vi "Actor Core.vi"(8 "error in":errorcluster, 11 "Nested in":refnum<class "CameraController.lvclass">) -> (0 "error out":errorcluster, 3 "Actor out":refnum<class "Actor.lvclass">)   [LabVIEW 2020, in "CameraController.lvlib" / "CameraController.lvclass"]
doc: "(<B>Filename</B>: Actor Framework.lvlib:Actor.lvclass:Actor Core.vi)\n\nReceives messages to the actor, reacts to them, and initiates any error handling that may shut the actor down.\n\nDescendant classes may override this VI to append parallel tasks for the actor to complete while it handles messages. Overrides use the Call Parent Method node."
uses:
  CameraController.lvclass
  <vilib>/ActorFramework/Actor/Actor.lvclass
  <vilib>/ActorFramework/Stop Msg/Stop Msg.lvclass
  C:/Program Files/National Instruments/LabVIEW 2020/vi.lib/ActorFramework/Actor/Actor.lvclass
  D:/Daguan/Development/MMicroscopyFramework/ViewController/Prime95BCameraController/CameraController.lvclass
  D:/Daguan/Development/MMicroscopyFramework/Interface/DataListener/DataListener.lvclass
  Model/Hardware Abstraction Layer/Component/Camera/Camera Messages/SetExposure Msg/SetExposure Msg.lvclass
  Model/Hardware Abstraction Layer/Component/Device/Device Messages/StopAcquisition Msg/StopAcquisition Msg.lvclass
  Model/Hardware Abstraction Layer/Component/Camera/Camera Messages/SetBinning Msg/SetBinning Msg.lvclass
  Interface/StageController Messages/SetStagePosition Msg/SetStagePosition Msg.lvclass
  Model/Hardware Abstraction Layer/Component/Camera/Camera Messages/SetFrameToCaptureNumber Msg/SetFrameToCaptureNumber Msg.lvclass
  Model/Hardware Abstraction Layer/Component/Camera/Camera Messages/SetInterval Msg/SetInterval Msg.lvclass
  CameraController Messages/PrepareAndSendROI Msg/PrepareAndSendROI Msg.lvclass
  Model/Hardware Layer/Real Hardware/Camera_Prime95B/Camera_Prime95B/Controls/Camera Status.ctl
  Model/Hardware Layer/Real Hardware/Camera_Prime95B/Camera_Prime95B/Camera_Prime95B.lvclass
  CameraController Messages/PrepareAndSendStartAcq Msg/PrepareAndSendStartAcq Msg.lvclass
panel:
  in  "Display?":bool
  in  "ThreadholdMin":i32=500
  in  "ROITool":bool
  in  "ZoomTool":bool
  in  "Autostretch":bool
  in  "ZoomToFit":bool
  in  "Save Path":path
  in  "Alert when finish?":bool
  in  "SingleStack?":bool
  in  "StreamToDisk?":bool
  in  "Binning":enum32{"1x1", "2x2"}(radio)
  in  "File Suffix":string
  in  "Full":bool
  in  "Crop":bool
  in  "Scale Bar":bool
  in  "ScaleBarSize":dbl caption="um" min=0.0 max=50.0
  in  "ThreadholdMax":u32(slide) max=4096 step=1 scale=0.0..10.0
  in  "Save Settings":bool
  in  "Snap":bool
  in  "Live":bool
  in  "Acquire":bool
  in  "Stop":bool
  in  "Album":bool
  in  "Exit":bool
  in  "Interval":dbl min=0.0 max=99999.0
  in  "Frames":dbl min=0.0 max=5000.0
  in  "ExposureMs":dbl min=0.0 max=99999.0
  out "DropFrames":dbl
  out "RealFPS":dbl
  out "ImgIndex":dbl
  out "RawImage":T1(plugin-control)
  # "ROI"
  # "Save Image Mode"
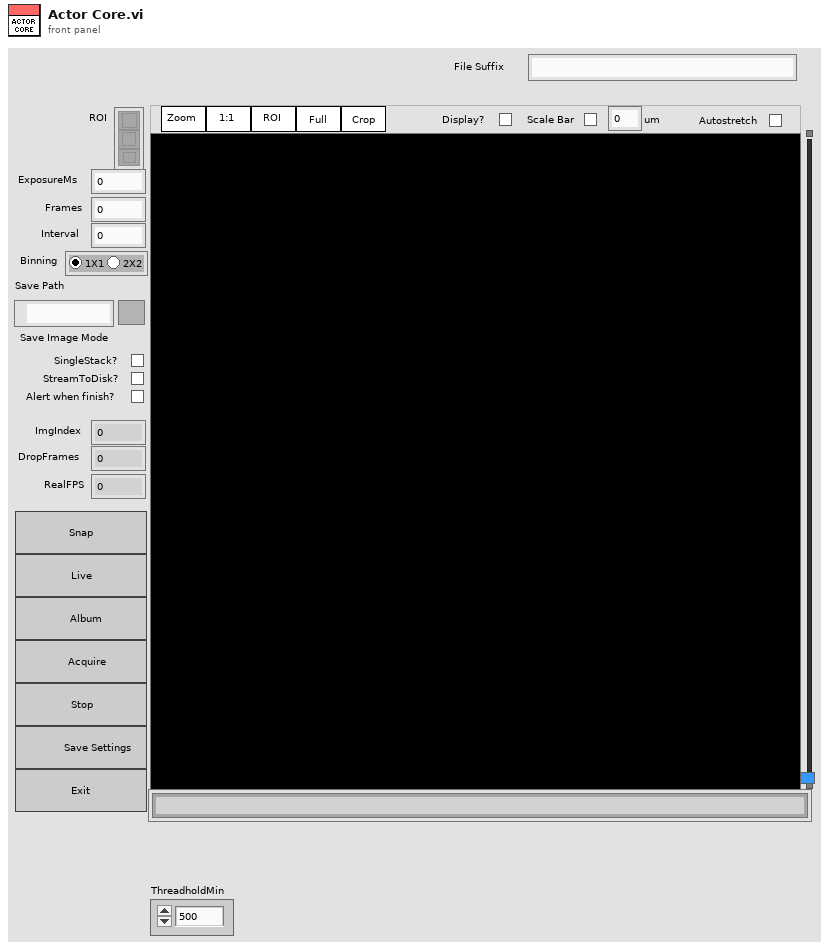
[diagram p1: front panel]
types:
  T1 = typedef "IMAQ Image.ctl" = refnum<image>
  T2 = cluster{"Stop":refnum<user-event>, "RawImage":refnum<user-event>}
  T3 = cluster{"Global Rectangle":i32[], "Contours":cluster{"Contour Type":u32, "ROI Type":u32, "Points":i32[]}[]}
  T4 = typedef "Camera_Prime95B.lvlib/Camera_Prime95B.lvclass/Camera Status.ctl" = i32
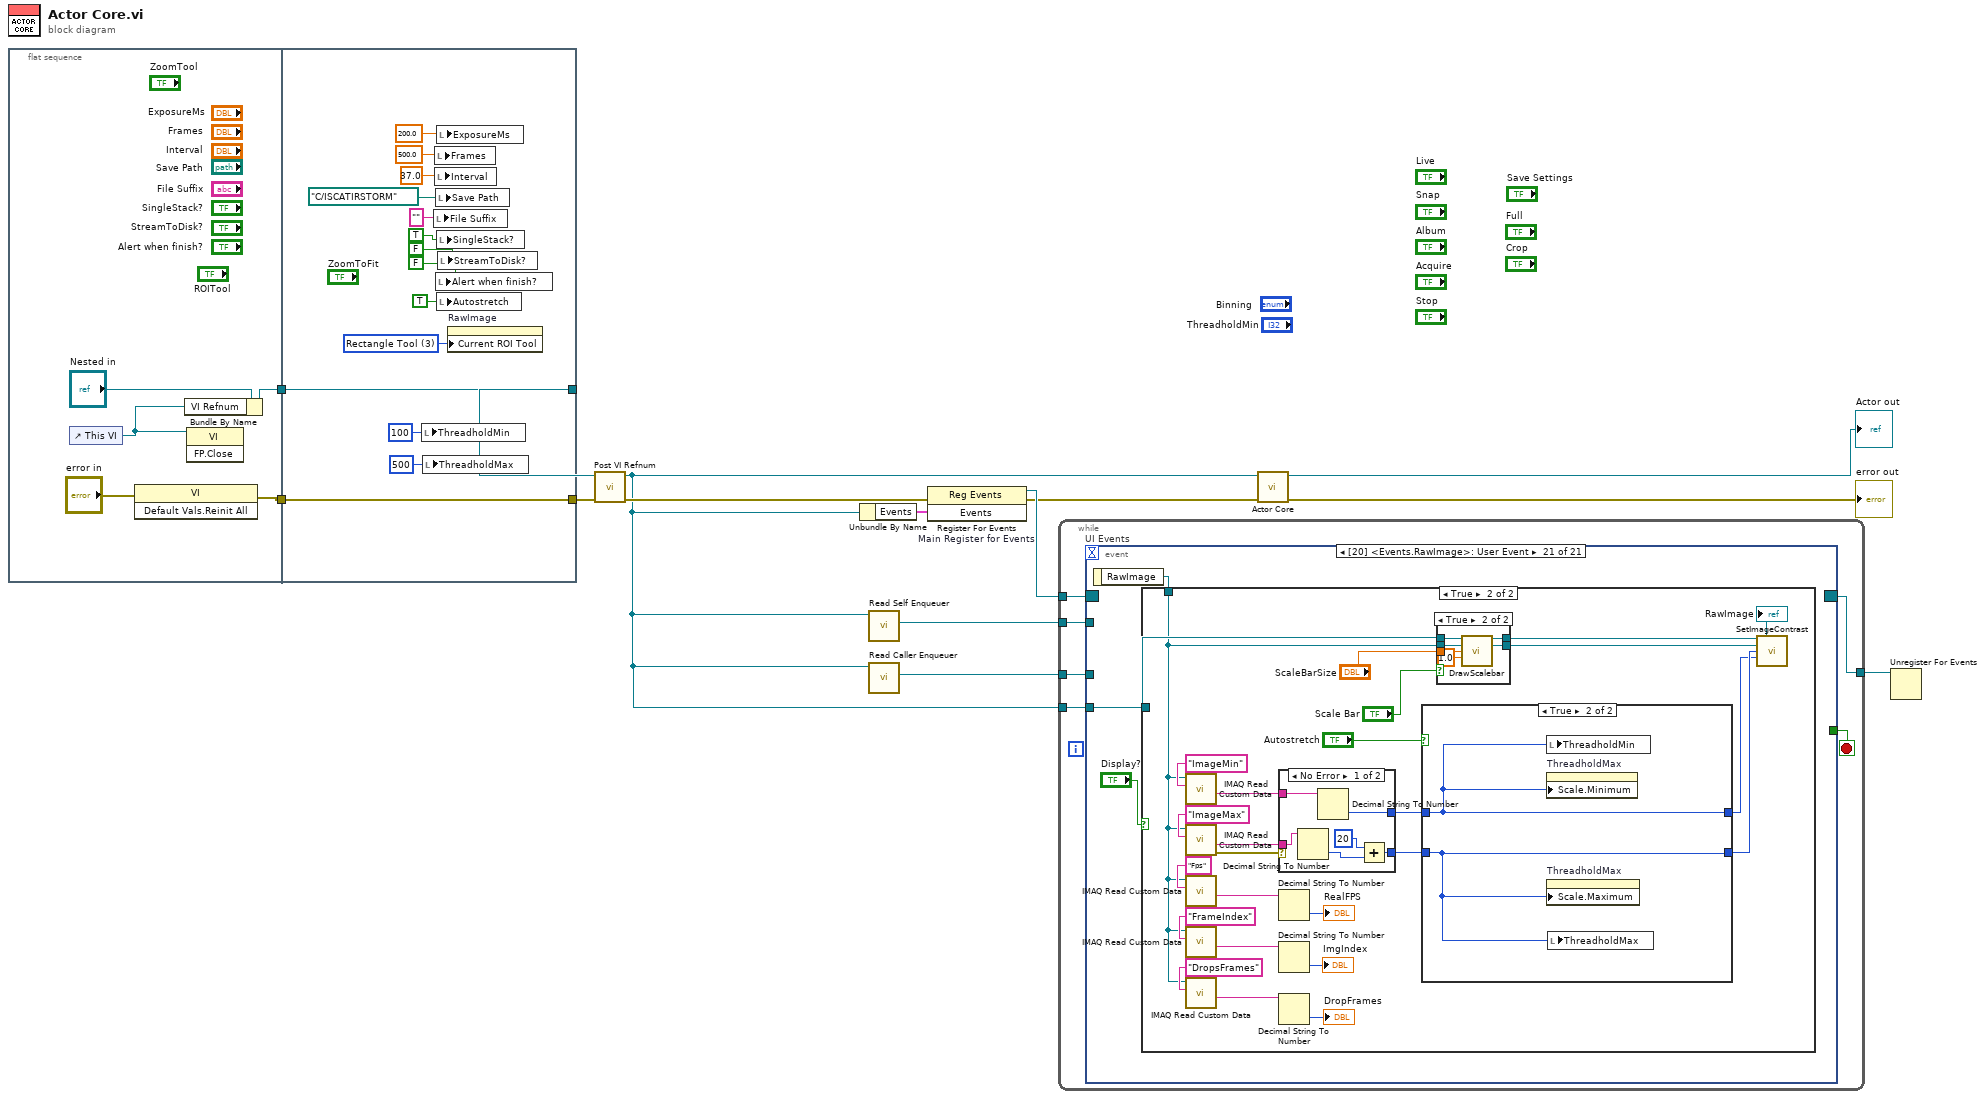
[diagram p0: block diagram]
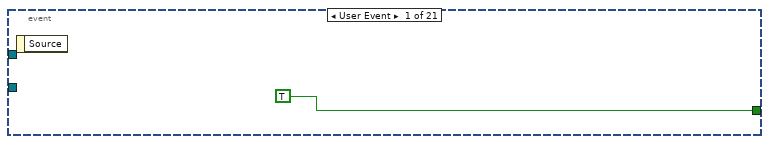
[diagram p2: hidden frame]
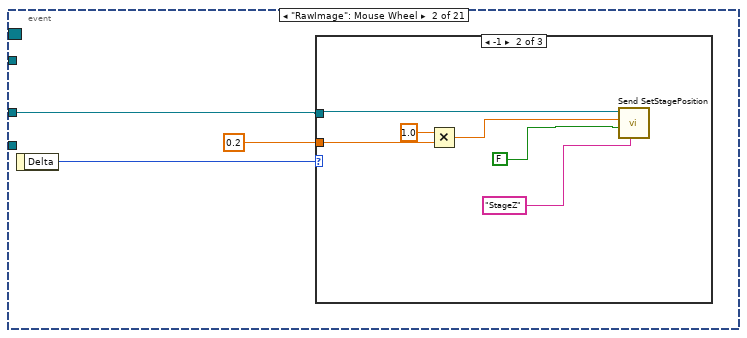
[diagram p3: hidden frame]
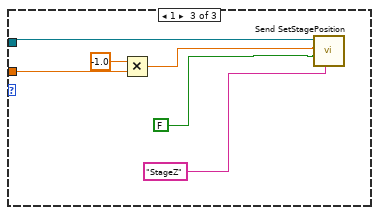
[diagram p5: hidden frame]
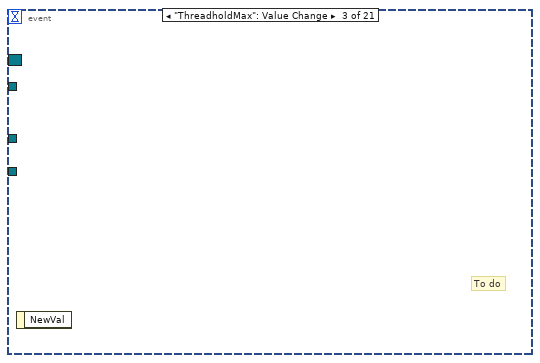
[diagram p6: hidden frame]
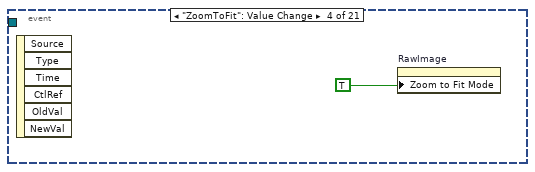
[diagram p7: hidden frame]
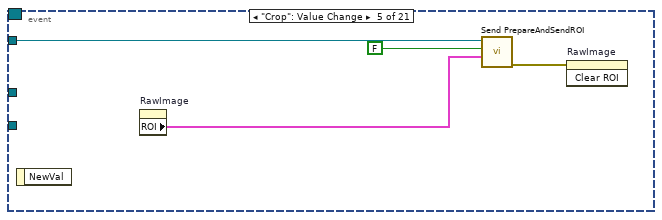
[diagram p8: hidden frame]
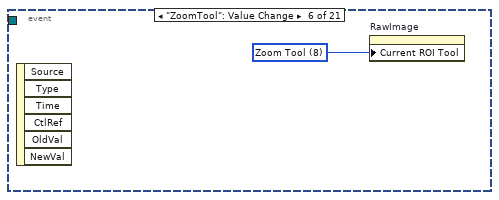
[diagram p9: hidden frame]
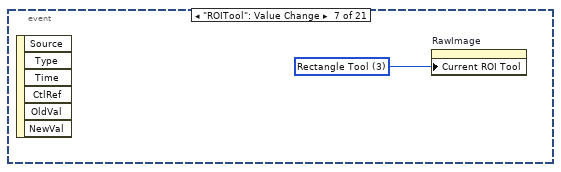
[diagram p10: hidden frame]
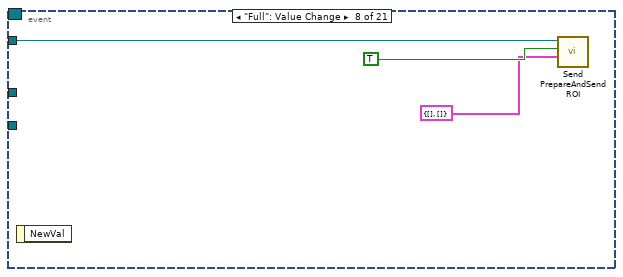
[diagram p11: hidden frame]
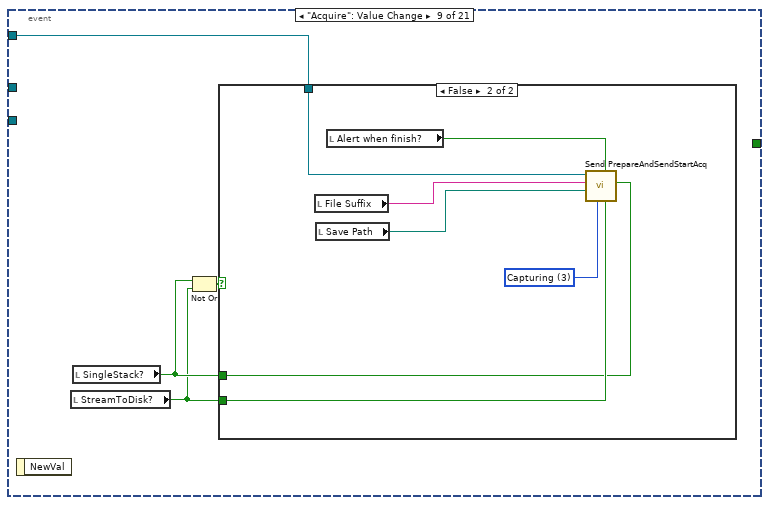
[diagram p12: hidden frame]
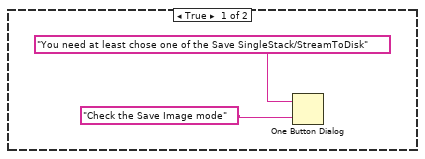
[diagram p13: hidden frame]
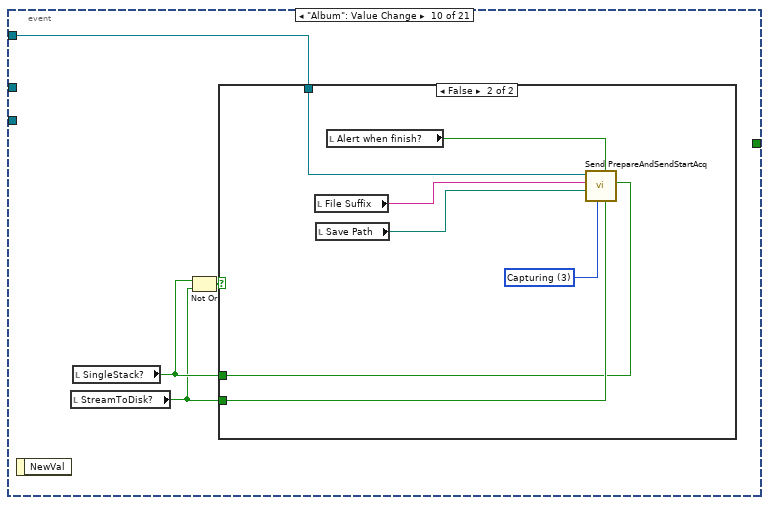
[diagram p14: hidden frame]
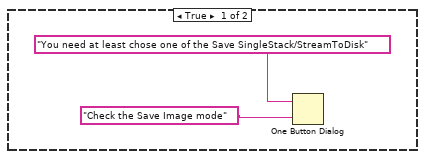
[diagram p15: hidden frame]
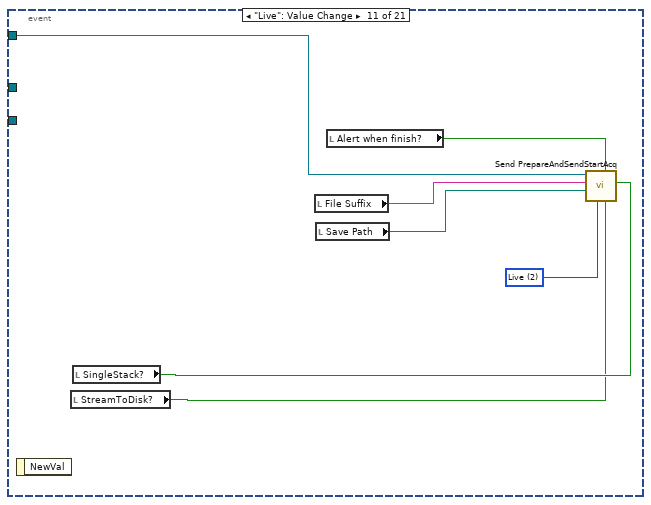
[diagram p16: hidden frame]
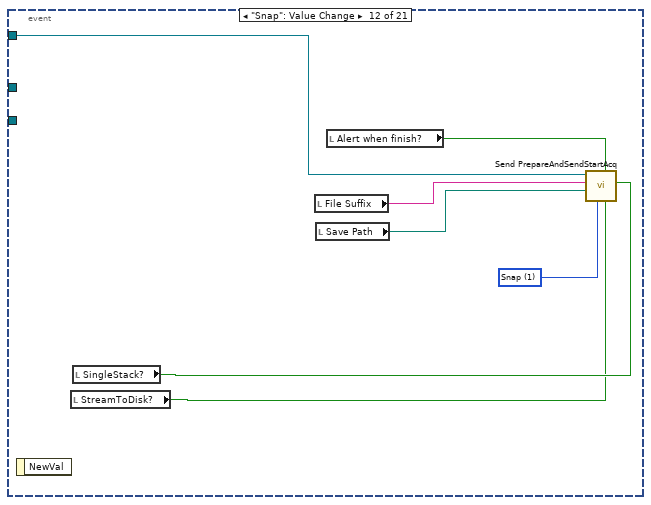
[diagram p17: hidden frame]
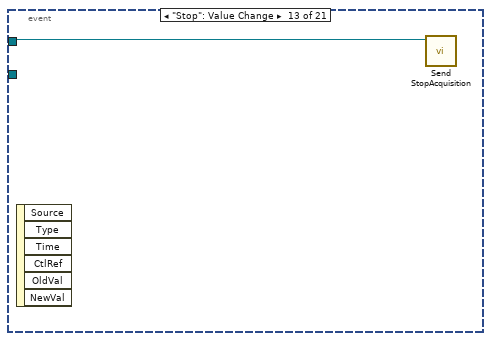
[diagram p18: hidden frame]
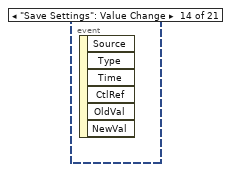
[diagram p19: hidden frame]
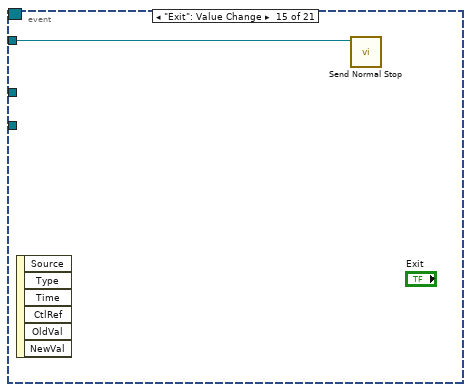
[diagram p20: hidden frame]
diagram:
  n1 = flat-sequence {
    tunnel: [w17] -> w6
    tunnel: [w16] -> w5
    tunnel: [w32] -> w2
    tunnel: [w33] -> w7
    tunnel: w6 -> [w33]
    tunnel: w5 -> [w32]
    frame #0 {
      n2 = control-ref of="This VI"() -> (w15:refnum<vi>)
      n3 = invoke class="VI" method="Default Vals.Reinit All"(error in="error in") -> (error out=w17:errorcluster)  [unwired: 2 in, 2 out]
      n4 = Bundle By Name(cluster="Nested in", "VI Refnum"=w15) -> (w16:refnum<class "CameraController.lvclass">)
      n5 = invoke class="VI" method="FP.Close"(reference=w15) -> ()  [unwired: 2 in, 3 out]
    }
    frame #1 {
      w23 = u32 3 items=["Zoom Tool"=8, "Selection Tool"=0, "Pan Tool"=9, "Point Tool"=1, "Line Tool"=2, "Rectangle Tool"=3, "Rotated Rectangle Tool"=12, "Polyline Tool"=10, "Polygon Tool"=5, "Freehand Tool"=11, "Closed Freehand Tool"=6, "Ellipse Tool"=4, "Annulus Tool"=7] ("Current ROI Tool")
      n6 = local write "ThreadholdMin"(100 ("ThreadholdMin")) -> ()
      n7 = local write "ThreadholdMax"(u32 500 ("ThreadholdMax")) -> ()
      n8 = local write "File Suffix"("" ("File suffix")) -> ()
      n9 = local write "Frames"(500.0 ("Frames")) -> ()
      n10 = local write "Interval"(37.0 ("Interval")) -> ()
      n11 = local write "Save Path"(path "C:/ISCATIRSTORM" ("Save Path")) -> ()
      n12 = local write "Alert when finish?"(FALSE ("Alert when finish?")) -> ()
      n13 = local write "ExposureMs"(200.0 ("ExposureMs")) -> ()
      n14 = local write "SingleStack?"(TRUE ("SingleStack?")) -> ()
      n15 = local write "Autostretch"(TRUE ("Autostretch")) -> ()
      n16 = local write "StreamToDisk?"(FALSE ("StreamToDisk?")) -> ()
      n17 = property on="RawImage" class="ImageControl"("Current ROI Tool"=w23) -> ()  [unwired: 2 in, 2 out]
    }
  }
  n18 = call-dynamic "Post VI Refnum.vi"("error in (no error)"=w7, "Camera Prime95B Controller in"=w2) -> ("error out"=w3:errorcluster, "Camera Prime95B Controller out"=w1:refnum<class "CameraController.lvclass">)  [unwired: 8 in]
  n19 = Unbundle By Name(w1) -> ("Events"=w11:T2)
  n20 = call <vilib>:"Read Self Enqueuer.vi"("Actor"=w1) -> ("Self Enqueuer"=w9:refnum<class "Message Enqueuer.lvclass">)  [unwired: 10 in]
  n21 = call <vilib>:"Read Caller Enqueuer.vi"("Actor"=w1) -> ("Caller Enqueuer"=w4:refnum<class "Message Enqueuer.lvclass">)  [unwired: 10 in]
  n22 = register-events "Main Register for Events"(error in=w3, w11) -> (reference out=w12:refnum<event-registration>, error out=w8:errorcluster)  [unwired: 1 in]
  n23 = while {
    tunnel: w12 -> [w39]
    tunnel: [w37] -> w10
    tunnel: w9 -> [w36]
    tunnel: w4 -> [w35]
    tunnel: w1 -> [w34]
    stop <- w38 stop-if-true
    n24 = event "UI Events" shown="[20] <Events.RawImage>: User Event" {
      selector: w39 -> [_ _ _ _ _ _ _ _ _ _ _ _ _ _ _ _ _ _ _ _ _]
      dyn-events: [_ _ _ _ _ _ _ _ _ _ _ _ _ _ _ _ _ _ _ _ _] -> w37
      timeout: _ -> [_ _ _ _ _ _ _ _ _ _ _ _ _ _ _ _ _ _ _ _ _]
      tunnel: [TRUE _ _ _ _ _ _ _ _ _ _ _ _ _ _ _ _ _ _ _ _] -> w38
      tunnel: w36 -> [_ _ _ _ w60 _ _ w65 w66 w79 w96 w103 _ _ w107 _ _ _ _ w117 _]
      tunnel: w35 -> [_ w42 _ _ _ _ _ _ _ _ _ _ w106 _ _ w109 w111 w113 w116 _ _]
      tunnel: w34 -> [_ _ _ _ _ _ _ _ _ _ _ _ _ _ _ _ _ _ _ _ w121]
      event User Event {
        n25 = event-data() -> ()  [unwired: 1 in, 1 out]
      }
      event "RawImage": Mouse Wheel {
        n26 = event-data() -> ("Delta"=w43:i32)  [unwired: 1 in]
        n27 = case shown="-1" w43 {
          tunnel: w42 -> [_ w47 w53]
          tunnel: 0.2 ("Value") -> [_ w49 w55]
          frame 0, Default {
          }
          frame -1 {
            n28 = Multiply(x=1.0, y=w49) -> (x*y=w46:dbl)
            n29 = call "Send SetStagePosition.vi"("Label"="StageZ" ("Message"), "AbsPosition?"=FALSE, "Value"=w46, "Message Enqueuer"=w47) -> ()  [unwired: 6 in, 2 out]
          }
          frame 1 {
            n30 = Multiply(x=-1.0, y=w55) -> (x*y=w52:dbl)
            n31 = call "Send SetStagePosition.vi"("Label"="StageZ" ("Message"), "AbsPosition?"=FALSE, "Value"=w52, "Message Enqueuer"=w53) -> ()  [unwired: 6 in, 2 out]
          }
        }
      }
      event "ThreadholdMax": Value Change {
        # "To do"
        n32 = event-data() -> ()  [unwired: 1 in, 1 out]
      }
      event "ZoomToFit": Value Change {
        n33 = event-data() -> ()  [unwired: 1 in, 6 out]
        n34 = property on="RawImage" class="ImageControl"("Zoom to Fit Mode"=TRUE) -> ()  [unwired: 2 in, 2 out]
      }
      event "Crop": Value Change {
        n35 = event-data() -> ()  [unwired: 1 in, 1 out]
        n36 = property on="RawImage" class="ImageControl"() -> ("ROI"=w58:T3)  [unwired: 2 in, 2 out]
        n37 = call "Send PrepareAndSendROI.vi"("ROI"=w58, "Clear ROI?(F)"=FALSE, "Message Enqueuer"=w60) -> ("error out"=w57:errorcluster)  [unwired: 7 in, 1 out]
        n38 = invoke on="RawImage" class="ImageControl" method="Clear ROI"(error in=w57) -> ()  [unwired: 2 in, 3 out]
      }
      event "ZoomTool": Value Change {
        w61 = u32 8 items=["Zoom Tool"=8, "Selection Tool"=0, "Pan Tool"=9, "Point Tool"=1, "Line Tool"=2, "Rectangle Tool"=3, "Rotated Rectangle Tool"=12, "Polyline Tool"=10, "Polygon Tool"=5, "Freehand Tool"=11, "Closed Freehand Tool"=6, "Ellipse Tool"=4, "Annulus Tool"=7] ("Current ROI Tool")
        n39 = event-data() -> ()  [unwired: 1 in, 6 out]
        n40 = property on="RawImage" class="ImageControl"("Current ROI Tool"=w61) -> ()  [unwired: 2 in, 2 out]
      }
      event "ROITool": Value Change {
        w62 = u32 3 items=["Zoom Tool"=8, "Selection Tool"=0, "Pan Tool"=9, "Point Tool"=1, "Line Tool"=2, "Rectangle Tool"=3, "Rotated Rectangle Tool"=12, "Polyline Tool"=10, "Polygon Tool"=5, "Freehand Tool"=11, "Closed Freehand Tool"=6, "Ellipse Tool"=4, "Annulus Tool"=7] ("Current ROI Tool")
        n41 = event-data() -> ()  [unwired: 1 in, 6 out]
        n42 = property on="RawImage" class="ImageControl"("Current ROI Tool"=w62) -> ()  [unwired: 2 in, 2 out]
      }
      event "Full": Value Change {
        n43 = event-data() -> ()  [unwired: 1 in, 1 out]
        n44 = call "Send PrepareAndSendROI.vi"("ROI"=T3 {"Global Rectangle"=[], "Contours"=[]}, "Clear ROI?(F)"=TRUE, "Message Enqueuer"=w65) -> ()  [unwired: 7 in, 2 out]
      }
      event "Acquire": Value Change {
        n45 = event-data() -> ()  [unwired: 1 in, 1 out]
        n46 = local read "StreamToDisk?"() -> (w68:bool)
        n47 = local read "SingleStack?"() -> (w69:bool)
        n48 = Not Or(1:w68, 2:w69) -> (0:w67:bool)
        n49 = case shown="False" w67 {
          tunnel: w69 -> [_ w72]
          tunnel: w68 -> [_ w74]
          tunnel: w66 -> [_ w78]
          frame True {
            n50 = One Button Dialog(message="You need at least chose one of the Save SingleStack/StreamToDisk", button name ("OK")="Check the Save Image mode" ("message")) -> ()  [unwired: 1 out]
          }
          frame False {
            w75 = T4 3 items=["Idle", "Snap", "Live", "Capturing", ""] ("Mode")
            n51 = local read "File Suffix"() -> (w77:string)
            n52 = local read "Save Path"() -> (w76:path)
            n53 = local read "Alert when finish?"() -> (w73:bool)
            n54 = call "Send PrepareAndSendStartAcq.vi"("SingleStack?"=w72, "StreamToDisk?"=w74, "Alert when finish?"=w73, "Mode"=w75, "Save Path"=w76, "File Suffix"=w77, "Message Enqueuer"=w78) -> ()  [unwired: 3 in, 2 out]
          }
        }
      }
      event "Album": Value Change {
        n55 = event-data() -> ()  [unwired: 1 in, 1 out]
        n56 = local read "StreamToDisk?"() -> (w81:bool)
        n57 = local read "SingleStack?"() -> (w82:bool)
        n58 = Not Or(1:w81, 2:w82) -> (0:w80:bool)
        n59 = case shown="False" w80 {
          tunnel: w82 -> [_ w85]
          tunnel: w81 -> [_ w87]
          tunnel: w79 -> [_ w91]
          frame True {
            n60 = One Button Dialog(message="You need at least chose one of the Save SingleStack/StreamToDisk", button name ("OK")="Check the Save Image mode" ("message")) -> ()  [unwired: 1 out]
          }
          frame False {
            w88 = T4 3 items=["Idle", "Snap", "Live", "Capturing", ""] ("Mode")
            n61 = local read "File Suffix"() -> (w90:string)
            n62 = local read "Save Path"() -> (w89:path)
            n63 = local read "Alert when finish?"() -> (w86:bool)
            n64 = call "Send PrepareAndSendStartAcq.vi"("SingleStack?"=w85, "StreamToDisk?"=w87, "Alert when finish?"=w86, "Mode"=w88, "Save Path"=w89, "File Suffix"=w90, "Message Enqueuer"=w91) -> ()  [unwired: 3 in, 2 out]
          }
        }
      }
      event "Live": Value Change {
        w93 = T4 2 items=["Idle", "Snap", "Live", "Capturing", ""] ("Mode")
        n65 = event-data() -> ()  [unwired: 1 in, 1 out]
        n66 = local read "StreamToDisk?"() -> (w97:bool)
        n67 = local read "SingleStack?"() -> (w98:bool)
        n68 = local read "File Suffix"() -> (w95:string)
        n69 = local read "Save Path"() -> (w94:path)
        n70 = local read "Alert when finish?"() -> (w92:bool)
        n71 = call "Send PrepareAndSendStartAcq.vi"("SingleStack?"=w98, "StreamToDisk?"=w97, "Alert when finish?"=w92, "Mode"=w93, "Save Path"=w94, "File Suffix"=w95, "Message Enqueuer"=w96) -> ()  [unwired: 3 in, 2 out]
      }
      event "Snap": Value Change {
        w100 = T4 1 items=["Idle", "Snap", "Live", "Capturing", ""] ("Mode")
        n72 = event-data() -> ()  [unwired: 1 in, 1 out]
        n73 = local read "StreamToDisk?"() -> (w104:bool)
        n74 = local read "SingleStack?"() -> (w105:bool)
        n75 = local read "File Suffix"() -> (w102:string)
        n76 = local read "Save Path"() -> (w101:path)
        n77 = local read "Alert when finish?"() -> (w99:bool)
        n78 = call "Send PrepareAndSendStartAcq.vi"("SingleStack?"=w105, "StreamToDisk?"=w104, "Alert when finish?"=w99, "Mode"=w100, "Save Path"=w101, "File Suffix"=w102, "Message Enqueuer"=w103) -> ()  [unwired: 3 in, 2 out]
      }
      event "Stop": Value Change {
        n79 = event-data() -> ()  [unwired: 1 in, 6 out]
        n80 = call "Send StopAcquisition.vi"("Message Enqueuer"=w106) -> ()  [unwired: 9 in, 2 out]
      }
      event "Save Settings": Value Change {
        n81 = event-data() -> ()  [unwired: 1 in, 6 out]
      }
      event "Exit": Value Change {
        n82 = event-data() -> ()  [unwired: 1 in, 6 out]
        n83 = call <vilib>:"Send Normal Stop.vi"("Message Enqueuer"=w107) -> ()  [unwired: 10 in, 1 out]
      }
      event "ExposureMs": Value Change {
        n84 = event-data() -> ("NewVal"=w108:dbl)  [unwired: 1 in]
        n85 = call "Send SetExposure.vi"("Setting.Exposure"=w108, "Message Enqueuer"=w109) -> ()  [unwired: 8 in, 2 out]
      }
      event "Frames": Value Change {
        n86 = event-data() -> ("NewVal"=w110:dbl)  [unwired: 1 in]
        n87 = call "Send SetFrameToCaptureNumber.vi"("Setting.FramesToCapture"=w110, "Message Enqueuer"=w111) -> ()  [unwired: 8 in, 2 out]
      }
      event "Interval": Value Change {
        n88 = event-data() -> ("NewVal"=w112:dbl)  [unwired: 1 in]
        n89 = call "Send SetInterval.vi"("Setting.Interval"=w112, "Message Enqueuer"=w113) -> ()  [unwired: 8 in, 2 out]
      }
      event "Binning": Value Change {
        n90 = event-data() -> ("NewVal"=w115:enum32{"1x1", "2x2"})  [unwired: 1 in]
        n91 = Increment(x=w115) -> (x+1=w114:enum32{"1x1", "2x2"})
        n92 = call "Send SetBinning.vi"("Setting.Binning.BinY"=w114, "Setting.Binning.BinX"=w114, "Message Enqueuer"=w116) -> ()  [unwired: 7 in, 2 out]
      }
      event Panel Close? {
        n93 = event-data() -> ()  [unwired: 1 in, 1 out]
        n94 = call <vilib>:"Send Normal Stop.vi"("Message Enqueuer"=w117) -> ()  [unwired: 10 in, 1 out]
        n95 = event-data("Discard?"=TRUE) -> ()  [unwired: 1 in, 1 out]
      }
      event User Event {
        n96 = event-data() -> ("RawImage"=w120:T1)  [unwired: 1 in]
        n97 = case shown="True" "Display?" {
          tunnel: w121 -> [_ w133]
          tunnel: w120 -> [_ w130]
          frame False {
          }
          frame True {
            n98 = call "IMAQ Read Custom Data"("Key"="ImageMin", "Image"=w130) -> ("Custom Data Out"=w128:string)  [unwired: 7 in, 2 out]
            n99 = call "IMAQ Read Custom Data"("Key"="ImageMax", "Image"=w130) -> ("error out"=w124:errorcluster, "Custom Data Out"=w129:string)  [unwired: 7 in, 1 out]
            n100 = call "IMAQ Read Custom Data"("Key"="Fps", "Image"=w130) -> ("Custom Data Out"=w144:string)  [unwired: 7 in, 2 out]
            n101 = call "IMAQ Read Custom Data"("Key"="FrameIndex", "Image"=w130) -> ("Custom Data Out"=w134:string)  [unwired: 7 in, 2 out]
            n102 = call "IMAQ Read Custom Data"("Key"="DropsFrames", "Image"=w130) -> ("Custom Data Out"=w143:string)  [unwired: 7 in, 2 out]
            n103 = case shown="No Error" w124 {
              tunnel: w129 -> [w153 _]
              tunnel: w128 -> [w152 _]
              tunnel: [w150 500] -> w125
              tunnel: [w151 0] -> w123
              frame No Error {
                n104 = Decimal String To Number(string=w153) -> (number=w149:i32)  [unwired: 2 in, 1 out]
                n105 = Decimal String To Number(string=w152) -> (number=w151:i32)  [unwired: 2 in, 1 out]
                n106 = Add(x=20, y=w149) -> (x+y=w150:i32)
              }
              frame Error {
              }
            }
            n107 = Decimal String To Number(string=w144) -> (number=→"RealFPS":i32)  [unwired: 2 in, 1 out]
            n108 = Decimal String To Number(string=w134) -> (number=→"ImgIndex":i32)  [unwired: 2 in, 1 out]
            n109 = Decimal String To Number(string=w143) -> (number=→"DropFrames":i32)  [unwired: 2 in, 1 out]
            n110 = case shown="True" "Autostretch" {
              tunnel: ["ThreadholdMax" w159] -> w126
              tunnel: w125 -> [_ w159]
              tunnel: w123 -> [_ w158]
              tunnel: [w156 w158] -> w122
              frame False {
                n111 = local read "ThreadholdMin"() -> (w156:i32)
              }
              frame True {
                n112 = local write "ThreadholdMin"(w158) -> ()
                n113 = property on="ThreadholdMax" class="Slide (strict)"("Scale.Minimum"=w158) -> ()  [unwired: 2 in, 2 out]
                n114 = property on="ThreadholdMax" class="Slide (strict)"("Scale.Maximum"=w159) -> ()  [unwired: 2 in, 2 out]
                n115 = local write "ThreadholdMax"(w159) -> ()
              }
            }
            n116 = case shown="True" "Scale Bar" {
              tunnel: w133 -> [w161 w167]
              tunnel: [w161 w166] -> w139
              tunnel: w130 -> [w160 w165]
              tunnel: [w160 w164] -> w138
              tunnel: "ScaleBarSize" -> [_ w163]
              frame False {
              }
              frame True {
                n117 = call-dynamic "DrawScalebar.vi"("CameraController in"=w167, "Image In"=w165, "ScaleBarSize"=w163, "Binning"=1.0) -> ("CameraController out"=w166:refnum<class "CameraController.lvclass">, "Image Out"=w164:T1)  [unwired: 9 in, 1 out]
              }
            }
            n118 = call-dynamic "SetImageContrast.vi"("CameraController in"=w139, "Image In"=w138, "Max"=w126, "Min"=w122) -> ("Image Dst Out"=→"RawImage":T1)  [unwired: 9 in, 2 out]
          }
        }
      }
    }
  }
  n119 = call-parent "Actor Core.vi"("error in"=w8, "Actor in"=w1) -> ("error out"=→"error out":errorcluster, "Actor out"=→"Actor out":refnum<class "Actor.lvclass">)  [unwired: 8 in]
  n120 = Unregister For Events(event registration refnum=w10) -> ()  [unwired: 1 in, 1 out]
